vi "Read Dew Point DBL.vi"(8 "error in":errorcluster, 10 "Source":string, 11 "Virtual Sensor from CSV in":refnum<class "Virtual Sensor from CSV.lvclass">) -> (0 "error out":errorcluster, 1 "Time Stamp":timestamp format="%<%x %.3X>T", 2 "Dew Point":dbl, 3 "Virtual Sensor from CSV out":refnum<class "Virtual Sensor from CSV.lvclass">)   [LabVIEW 2024, in "Virtual Sensor from CSV.lvclass"]
uses:
  Virtual Sensor from CSV.lvclass
  Virtual Sensor from CSV.lvclass/Virtual Sensor from CSV.ctl
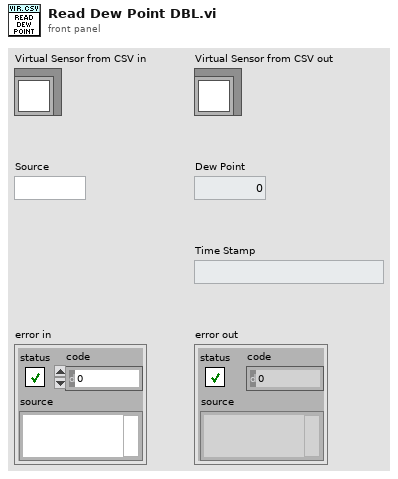
[diagram p1: front panel]
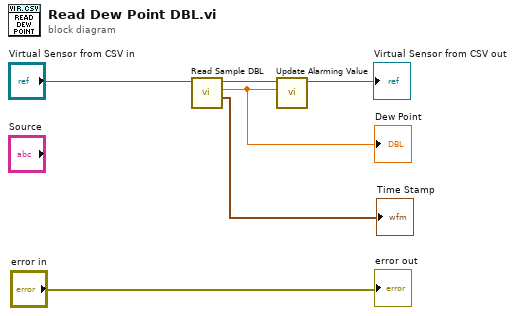
[diagram p0: block diagram]
diagram:
  n1 = call-dynamic "Read Sample DBL.vi"("Virtual Sensor from CSV in"="Virtual Sensor from CSV in") -> ("Time Stamp"=→"Time Stamp":timestamp, "Sample DBL"=w2:dbl, "Virtual Sensor from CSV out"=w3:refnum<class "Virtual Sensor from CSV.lvclass">)  [unwired: 8 in]
  "Dew Point" <- w2
  n2 = call "Update Alarming Value.vi"("Sample DBL"=w2, "Virtual Sensor from CSV in"=w3) -> ("Virtual Sensor from CSV out"=→"Virtual Sensor from CSV out":refnum<class "Virtual Sensor from CSV.lvclass">)  [unwired: 9 in]
  "error out" <- "error in"
